vi "_Register Menu Events.vi"(8 "error in (no error)":errorcluster, 9 "Menu Event":T1, 10 "Index":i32, 11 "Item_Refnums_Array":T2[](array[typedef])) -> (0 "error out":errorcluster, 3 "Item_Refnums_Array Out":T2[](array[typedef]))   [LabVIEW 2013, in "UI Panels.lvlib" / "Panels_XControl.xctl"]
uses:
  Panels_XControl.xctl
  Controls/References/Panel_Refnums.ctl
  Controls/Panel_Command_Enum.ctl
  Typedefs/Menu Event.ctl
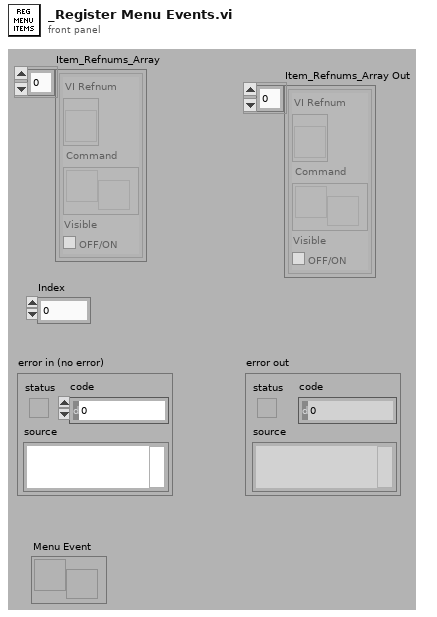
[diagram p1: front panel]
types:
  T1 = typedef "UI Panels.lvlib/Panels_XControl.xctl/Menu Event.ctl" = refnum<user-event>
  T2 = typedef "UI Panels.lvlib/Panels_XControl.xctl/Panel_Refnums.ctl" = cluster{"VI Refnum":refnum<vi>, "Command":refnum<user-event>, "Visible":bool}
  T3 = typedef "UI Panels.lvlib/Panels_XControl.xctl/Panel_Command_Enum.ctl" = enum16{"Idle", "Remove & Stop", "Add Item", "Delete Item", "Delete All", "Insert into Subpanel", "Register Menu Events", "Update Value", "Remove from Subpanel", "Set Title", "Set Menu Items", "Insert SubPanel", "Set Splitter Position", "Set Splitter Properties", "Add Menu Items"}
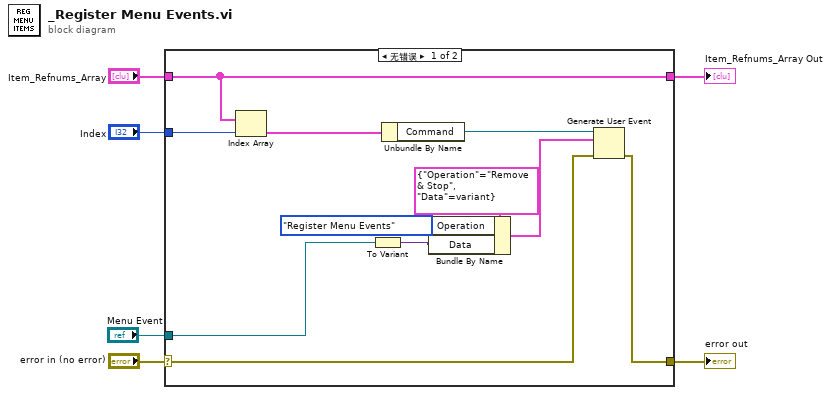
[diagram p0: block diagram]
diagram:
  n1 = case shown="无错误" "error in (no error)" {
    selector: "error in (no error)" -> [w8 w19]
    tunnel: "Index" -> [w15 _]
    tunnel: "Item_Refnums_Array" -> [w7 w18]
    tunnel: "Menu Event" -> [w12 _]
    tunnel: [w9 w19] -> w4
    tunnel: [w7 w18] -> w2
    frame No Error {
      n2 = Index Array(array=w7, index=w15) -> (element=w14:T2)
      n3 = To Variant(anything=w12) -> (Variant=w13:variant)
      n4 = Unbundle By Name(w14) -> ("Command"=w11:refnum<user-event>)
      n5 = Bundle By Name(cluster=cluster{"Operation":T3, "Data":variant} {"Operation"=enum."Remove & Stop", "Data"=variant} ("Item_Command"), "Operation"=Panel_Command_Enum."Register Menu Events", "Data"=w13) -> (w10:cluster{"Operation":T3, "Data":variant})
      n6 = Generate User Event(user event=w11, event data cluster=w10, error in=w8) -> (error out=w9:errorcluster)  [unwired: 1 in, 1 out]
    }
    frame Error {
    }
  }
  "Item_Refnums_Array Out" <- w2
  "error out" <- w4
